vi "Tool Q LEIN stroke fb value ovveride new.vi"(1 "Retry on err (F)":bool, 5 "stroke value(mm)":dbl, 7 "Pos Change":bool, 9 "Serial number(any number(-1))":i16=-1, 11 "error in (no error)":errorcluster, 12 "Solenoid 3":T1=3 items=["Don't change"=3, "On"=1, "Off"=2, "Unknown"=0], 13 "Solenoid 2":T1=3 items=["Don't change"=3, "On"=1, "Off"=2, "Unknown"=0], 14 "Solenoid 1":T1=3 items=["Don't change"=3, "On"=1, "Off"=2, "Unknown"=0]) -> (15 "error out":errorcluster)   [LabVIEW 2011]
doc: "-1 = any address:\n-2 = do not update"
uses:
  GUI/Tool detail view/Solenoid Status Override.ctl
  LEINmaster/Defenitions/LEIN Structure variations.ctl
  Application Structure/Options/Action GFV Settings.ctl
panel:
  # "-1 = any address:\n-2 =  do not update"
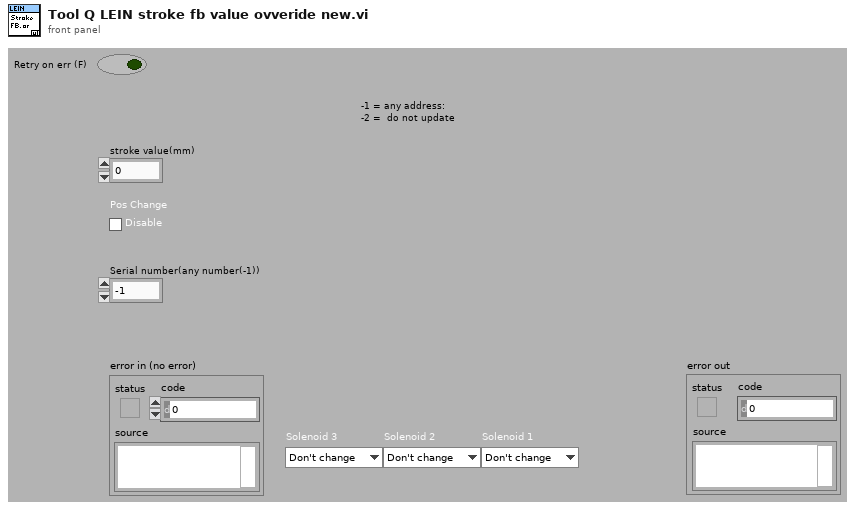
[diagram p1: front panel]
types:
  T1 = typedef "Solenoid Status Override.ctl" = u8
  T2 = typedef "Action GFV Settings.ctl" = enum16{"Init", "Get From INI", "Put In INI", "Get Settings", "Get Update Index", "Set Setting"}
  T3 = typedef "LEIN Structure variations.ctl" = enum16{"LEIN08", "LEIN31", "LEIN63"}
  T4 = enum16{"big-endian, network order", "native, host order", "little-endian"}
  T5 = typedef "Options  All pages and custom.ctl" = cluster{"P 1 (App)":T6, "P 2":T7, "P 3":T8, "P 4":T11, "P 5":T16, "P 6 (Err)":T17, "P 7 (Expert)":T18, "P 8 (Depth)":T20, "C 1":T21, "C 2":T22}
  T6 = typedef "Options Page 1 (App).ctl" = cluster{"Result files":path, "PCP Interface":string, "Tractor/Stroker Interface":string, "Tractor Interface":string, "Modem Status Interface":string, "Audible Alarm":bool, "Force alarm on Technical":bool, "Force alarm on HH":bool, "Force alarm on LL":bool, "Force alarm on H":bool, "Force alarm on L":bool}
  T7 = typedef "Options Page 2.ctl" = cluster{"Solenoid & Relay latching time":u16, "Tractor relay 1":dbl, "Tractor relay 2":dbl, "Tractor Solenoid limit":dbl}
  T8 = typedef "Options Page 3.ctl" = cluster{"Min resistance":dbl, "Max resistance":dbl, "Head voltage range":T9, "Max voltage jump":dbl, "Maximum resistance change":dbl, "Start Telemetry Voltage":dbl, "Start Telemetry Timeout":dbl, "Start Motor Voltage":dbl, "Stop Motor Voltage":dbl, "Pass Mode Warning Voltage":dbl, "Relay Switch Voltage":dbl, "Relay Status Loss Voltage":dbl, "Samples to average":i32, "PSU type DO NOT USE":T10, "Magna OVP":dbl, "Magna Current Limit":dbl}
  T9 = typedef "PCP type List.ctl" = enum16{"0 - 350V", "0 - 450V", "0 - 600V"}
  T10 = typedef "PSU Type.ctl" = enum16{"Unipower", "Magna 8.3A", "Magna 12A", "None"}
  T11 = typedef "Options Page 4.ctl" = cluster{"Solenoid & Relay latching time":u16, "Stroker relay 1":dbl, "Stroker Relay 2":dbl, "Stroker Solenoid limit":dbl, "Force det.":T12, "Stroke force lim.":dbl, "Anchor Enabled Pressure":dbl, "Tacometer puls":dbl, "Default anchor behavior":T13, "Default stroker behavior":T14, "Default stroker force limit (tonne)":dbl, "Slips Size":T15}
  T12 = typedef "Stroke force selector.ctl" = enum16{"Stroke in = node 1", "Strok out = node 1"}
  T13 = typedef "Default anchor behavior.ctl" = enum16{"Do nothing", "Set Anchor", "Release Anchor"}
  T14 = typedef "Default stroker behavior.ctl" = enum16{"Do nothing", "Stop", "Go Out", "Go In"}
  T15 = typedef "Slips Type Radio.ctl" = enum32{"No Selection", "338 MRS", "3,9 MRS"}
  T16 = typedef "Options Page 5.ctl" = cluster{"Solenoid & Relay latching time":u16, "Driller relay 1":dbl, "Driller Relay 2":dbl, "Driller  Solenoid limit":dbl}
  T17 = typedef "Options Page 6 (Err).ctl" = cluster{"Error and event files":path}
  T18 = typedef "Options Page 7 (Expert).ctl" = cluster{"Show Debug":bool, "Log debug messages":bool, "Additional debug messages":bool, "Start Beagle with Simulator data":bool, "Workshop mode":bool, "Modem baud":u16, "enumCANCOM":bool, "Modem sim":T19, "Telemetry Timeout Disable":i32, "Buffer size":i32, "Upd regular data":bool, "Cable comp":cluster{"VMOD1 Voltage(V)":dbl, "VMOD2 Voltage(V)":dbl}}
  T19 = typedef "Modem simulation setup.ctl" = cluster{"Modem dealay sim":bool, "Sim baud Tx":u16, "Bit Error fraction Tx":dbl, "Sim baud Rx":u16, "Bit Error fraction Rx":dbl}
  T20 = typedef "Options Page 8 (Depth).ctl" = cluster{"Winch Spool Circumference":dbl, "Winch Pulses per Revolution":dbl, "Current Depth":dbl}
  T21 = typedef "Options Custom 1.ctl" = cluster{"Depth Updated":bool, "Depth Offset":dbl}
  T22 = typedef "Options Custom 2.ctl" = cluster{"Placeholder":bool}
  T23 = typedef "LEIN CMD Cluster.ctl" = cluster{"SID":u8, "ANF":bool, "CMD":T24, "DATA":u8[]}
  T24 = typedef "LEIN CMD List.ctl" = enum8{"ACTI", "TASK", "RES0", "STAT", "RES1", "RES2", "RES3", "USER"}
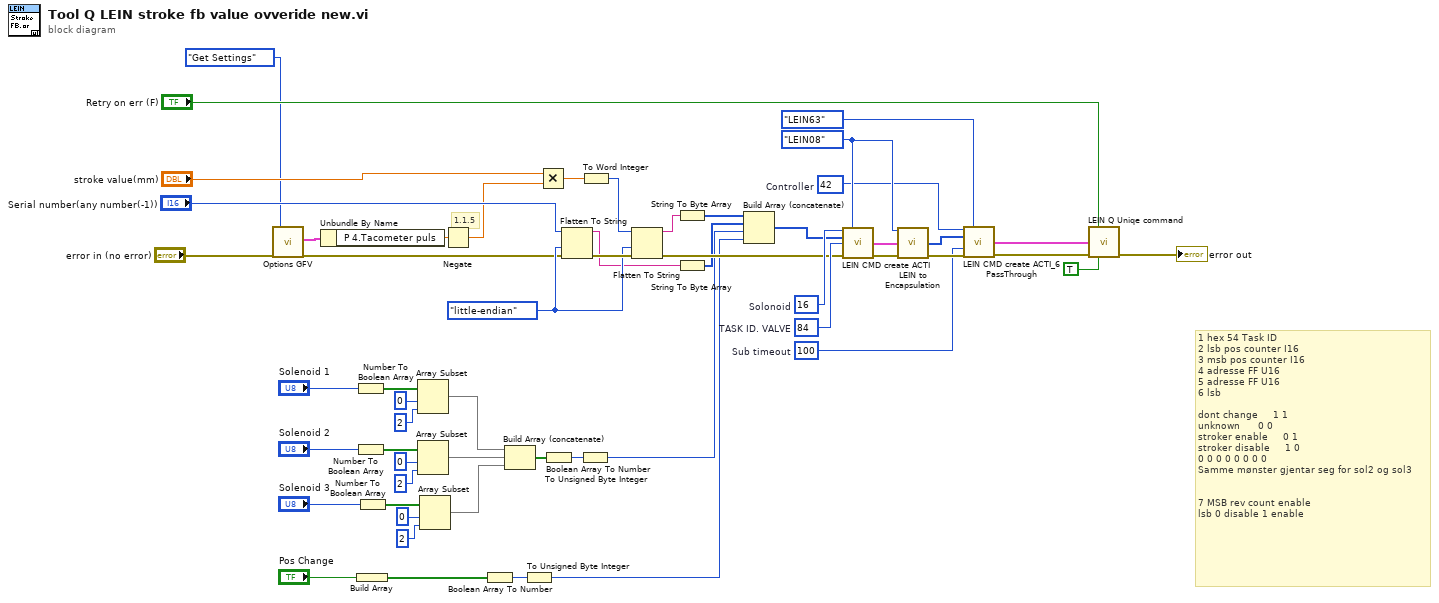
[diagram p0: block diagram]
diagram:
  w38 = u8 42  # Controller
  w39 = u8 16  # Solonoid
  w45 = u16 100  # Sub timeout
  w42 = u8 84  # TASK ID. VALVE
  w41 = LEIN_Structure_variations."LEIN08" ("LEIN Variation")
  w32 = T4."little-endian" ("byte order (0:big-endian, network order)")
  # "1 hex 54 Task ID\n2 lsb pos counter I16\n3 msb pos counter I16\n4 adresse FF U16\n5 adresse FF U16\n6 lsb \n\ndont change\t\t\t\t\t1\t1\nunknown\t\t\t\t\t\t0\t0\t\nstroker enable\t\t\t\t\t0\t1\nstroker disable\t\t\t\t\t1\t0\n0\t0\t0\t0\t0\t0\t0\t0\nSamme mønster gjentar seg for sol2 og sol3\n\n\n7 MSB rev count enable\nlsb 0 disable\t1 enable"
  # "1.1.5"
  n1 = call "Options GFV.vi"("error in (no error)"="error in (no error)", "Action(Get Settings)"=Action_GFV_Settings."Get Settings") -> ("Options"=w25:T5, "error out"=w26:errorcluster)  [unwired: 15 in, 1 out]
  n2 = Unbundle By Name(w25) -> ("P 4.Tacometer puls"=w24:dbl)
  n3 = Number To Boolean Array(number="Solenoid 1") -> (Boolean array=w20:bool[])
  n4 = Number To Boolean Array(number="Solenoid 2") -> (Boolean array=w21:bool[])
  n5 = Build Array("Pos Change") -> (w2:bool[])
  n6 = Number To Boolean Array(number="Solenoid 3") -> (Boolean array=w22:bool[])
  n7 = Array Subset(array=w20, index=0, length=2) -> (w10:bool[])
  n8 = Array Subset(array=w21, index=0, length=2) -> (w11:bool[])
  n9 = Array Subset(array=w22, index=0, length=2) -> (w12:bool[])
  n10 = Negate(x=w24) -> (-x=w23:dbl)
  n11 = Boolean Array To Number(Boolean array=w2) -> (number=w4:u32)
  n12 = Build Array (concatenate)(w10, w11, w12) -> (w13:bool[])
  n13 = To Unsigned Byte Integer(number=w4) -> (unsigned 8bit integer=w1:u8)
  n14 = Multiply(x="stroke value(mm)", y=w23) -> (x*y=w54:dbl)
  n15 = Boolean Array To Number(Boolean array=w13) -> (number=w6:u32)
  n16 = Flatten To String(anything="Serial number(any number(-1))", byte order (0:big-endian, network order)=w32, error in (no error)=w26) -> (data string=w30:string, error out=w33:errorcluster)  [unwired: 1 in, 1 out]
  n17 = To Unsigned Byte Integer(number=w6) -> (unsigned 8bit integer=w5:u8)
  n18 = To Word Integer(number=w54) -> (16bit integer=w53:i16)
  n19 = Flatten To String(anything=w53, byte order (0:big-endian, network order)=w32, error in (no error)=w33) -> (data string=w52:string, error out=w35:errorcluster)  [unwired: 1 in, 1 out]
  n20 = String To Byte Array(string=w52) -> (unsigned byte array=w40:u8[])
  n21 = String To Byte Array(string=w30) -> (unsigned byte array=w29:u8[])
  n22 = Build Array (concatenate)(w40, w29, w5, w1) -> (w34:u8[])
  n23 = call "LEIN CMD create ACTI.vi"("SID"=w39, "LEIN Variation"=w41, "Data"=w34, "ACTI ID"=w42, "error in (no error)"=w35) -> ("CMD"=w43:T23, "error out"=w44:errorcluster)  [unwired: 9 in]
  n24 = call "LEIN to Encapsulation.vi"("LEIN Variation"=w41, "CMD"=w43, "error in (no error)"=w44) -> ("Data and header"=w48:u8[], "error out"=w49:errorcluster)  [unwired: 8 in, 3 out]
  n25 = call "LEIN CMD create ACTI_6 PassThrough.vi"("SID"=w38, "LEIN Variation"=LEIN_Structure_variations."LEIN63", "LEIN ecapsulated data (header and data)"=w48, "Sub Timeout (ms)"=w45, "error in (no error)"=w49) -> ("CMD"=w47:T23, "error out"=w46:errorcluster)  [unwired: 9 in]
  n26 = call "LEIN Q Uniqe command.vi"("Retry on err (F)"="Retry on err (F)", "CMD"=w47, "error in"=w46, "priority(F)"=TRUE) -> ("error out"=→"error out":errorcluster)  [unwired: 11 in]
